vi "CSM - Delete Module Attribute.vi"(0 "CSM Name":string, 5 "Attribute":string, 9 "Wait (5000 ms)":i32=5000, 11 "Error In":errorcluster caption="error in (no error)") -> (4 "CSM Name (Dup)":string, 6 "Found":bool, 10 "Waited (ms)":u32, 15 "error out":errorcluster)   [LabVIEW 2017, in "Communicable State Machine.lvlib"]
uses:
  Communicable State Machine.lvlib
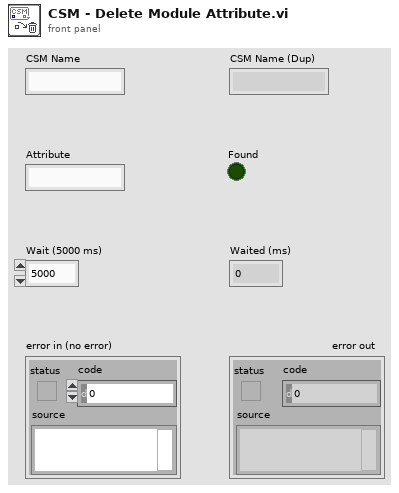
[diagram p1: front panel]
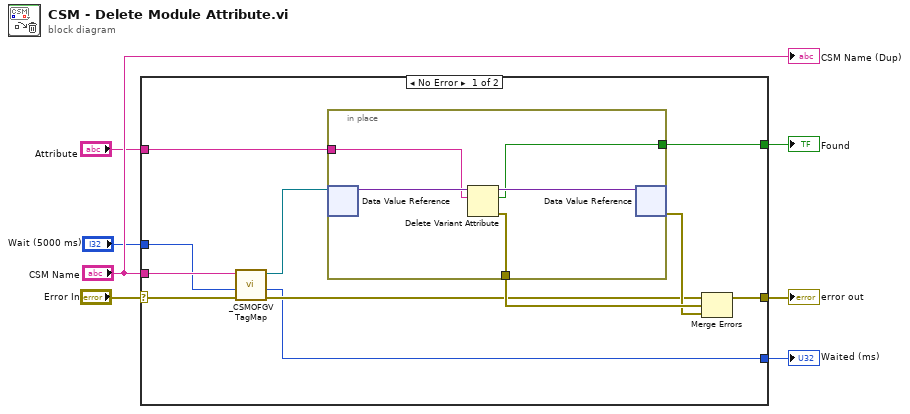
[diagram p0: block diagram]
diagram:
  n1 = case shown="No Error" "Error In" {
    selector: "Error In" -> [w12 w24]
    tunnel: [w16 w24] -> w6
    tunnel: "CSM Name" -> [w11 _]
    tunnel: "Attribute" -> [w15 _]
    tunnel: [w14 _] -> w3
    tunnel: "Wait (5000 ms)" -> [w10 _]
    tunnel: [w9 _] -> w1
    frame No Error {
      n2 = call "_CSMOFGV TagMap.vi"("error in (no error)"=w12, "Wait (5000 ms)"=w10, "CSM Name"=w11) -> ("error out"=w13:errorcluster, "Waited (ms)"=w9:u32, "TagMap"=w8:refnum<data-value>)  [unwired: 6 in]
      n3 = in-place {
        in-place-border: [w22] -> w18
        in-place-border: w15 -> [w21]
        in-place-border: [w19] -> w14
        n4 = in-place-dvr #1(w8) -> (w23:variant)  [unwired: 1 out]
        n5 = Delete Variant Attribute(6:w21, 7:w23) -> (0:w22:errorcluster, 2:w19:bool, 3:w20:variant)  [unwired: 1 in]
        n6 = in-place-dvr #1(w20) -> (w17:errorcluster)  [unwired: 1 out]
      }
      n7 = Merge Errors(w13, w18, w17) -> (w16:errorcluster)
    }
    frame Error {
    }
  }
  "error out" <- w6
  "Found" <- w3
  "Waited (ms)" <- w1
  "CSM Name (Dup)" <- "CSM Name"
